vi "ReadAttributeFrontPanelInMem.vi"(0 "reference in":refnum<class "G#MethodTemplates.lvclass">, 5 "error in (no error)":errorcluster) -> (14 "reference out":refnum<class "G#MethodTemplates.lvclass">, 19 "error out":errorcluster)   [LabVIEW 2020, in "G#MethodTemplates.lvclass"]
uses:
  G#MethodTemplates.lvclass
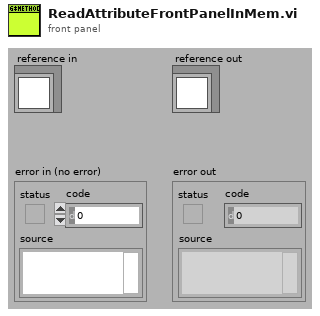
[diagram p1: front panel]
types:
  T1 = typedef "G#MethodTemplates.lvclass/ObjectAttributes.ctl" = cluster{"Numeric":dbl}
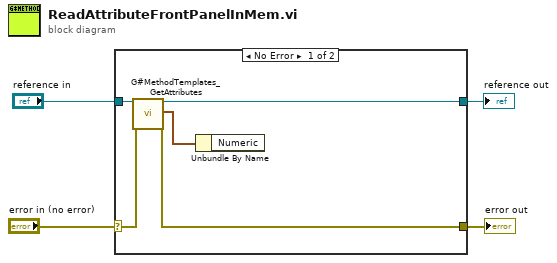
[diagram p0: block diagram]
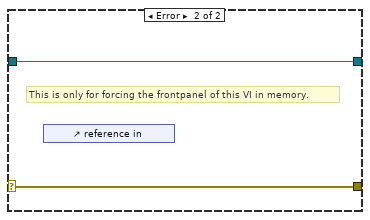
[diagram p2: hidden frame]
diagram:
  n1 = case shown="No Error" "error in (no error)" {
    selector: "error in (no error)" -> [w9 w11]
    tunnel: [w8 w11] -> w3
    tunnel: [w7 w10] -> w1
    tunnel: "reference in" -> [w5 w10]
    frame No Error {
      n2 = call "G#MethodTemplates_GetAttributes.vi"("reference in"=w5, "error in (no error)"=w9) -> ("reference out"=w7:refnum<class "G#MethodTemplates.lvclass">, "attributes"=w6:T1, "error out"=w8:errorcluster)  [unwired: 14 in, 1 out]
      n3 = Unbundle By Name(w6) -> ()  [unwired: 1 out]
    }
    frame Error {
      # "This is only for forcing the frontpanel of this VI in memory."
      n4 = control-ref of="reference in"() -> ()  [unwired: 1 out]
    }
  }
  "error out" <- w3
  "reference out" <- w1
